vi "PC_Main.vi"() -> ()   [LabVIEW 2020]
doc: "Use this template to build a producer/consumer design pattern with events to produce queue items. Use this design pattern instead of the User Interface Event Handler pattern for user interfaces when you want to execute code asynchronously in response to an event without slowing the user interface responsiveness."
uses:
  <vilib>/userdefined/High Color/nirio_resource_hc.ctl
  Invoked_events.ctl
  <vilib>/FPGAPlugInAG/Dynamic/niLvFpga_Close_Dynamic.vi
  <vilib>/FPGAPlugInAG/cRIO-9040/niLvFpga_Open_cRIO-9040.vi
  <vilib>/rvi/interface/common/dynamic/niFpgaDynamicAddResources.vi
  <vilib>/rvi/interface/nirviCloseFPGA/nirviCloseFPGA.xnode
  <vilib>/rvi/interface/nirviOpenFPGA/nirviOpenFPGA.xnode
  FPGA Bitfiles/depapp_FPGATarget_FPGAmain_WC8wSYHNwdY.lvbitx
  FPGA_main.vi
  <instrlib>/Siglent SDG 1000 5000 800 Series/Siglent SDG 1000 5000 800 Series.lvlib
panel:
  in  "Siglent Channel Control":enum32{"Channel 1", "Channel 2"}(tab)
  in  "Output Channel 1 Button":bool
  in  "Channel 1 Parameters":T1={"Peak-to-Peak Amplitude (V)"=0.1, "Frequency (Hz)"=1000.0, "DC Offset ( V)"=0.0, "Waveform Function (0: Sine)"=enum."Sine"} caption="Cluster"
  in  "Channel 2 Parameters":T1={"Peak-to-Peak Amplitude (V)"=0.1, "Frequency (Hz)"=1000.0, "DC Offset ( V)"=0.0, "Waveform Function (0: Sine)"=enum."Sine"} caption="Cluster"
  in  "Output Channel 2 Button":bool
  in  "resource name":T2
  out "FPGA VI Reference Out":refnum<k20>
  in  "Siglent Resource Name":refnum<visa-resource-name>
  in  "Siglent":bool
  in  "FPGA":bool
  in  "stop":bool
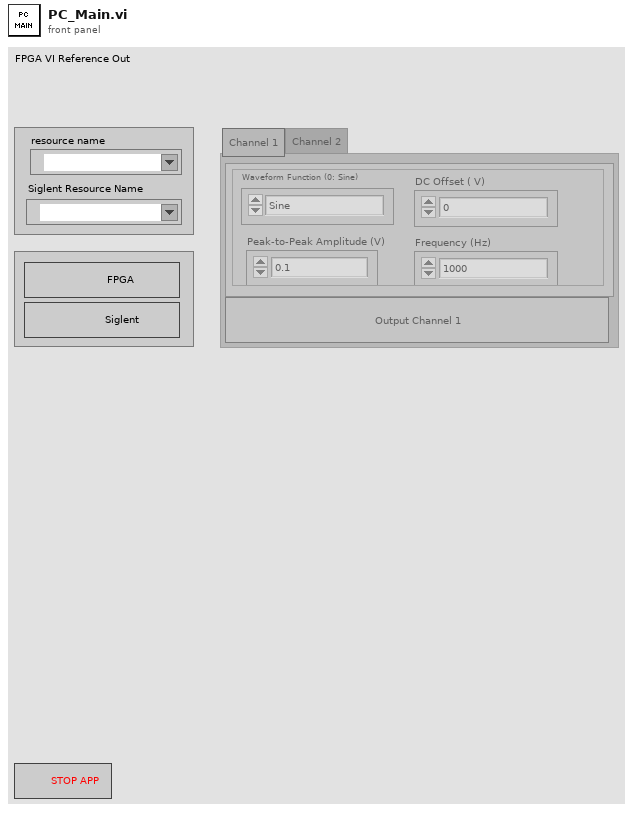
[diagram p1: front panel]
types:
  T1 = cluster{"Peak-to-Peak Amplitude (V)":dbl, "Frequency (Hz)":dbl, "DC Offset ( V)":dbl, "Waveform Function (0: Sine)":enum16{"Sine", "Square", "Triangle", "DC", "Pulse", "Arb"}}
  T2 = typedef "nirio_resource_hc.ctl" = tag
  T3 = typedef "Invoked_events.ctl" = enum16{"Siglent Channel Output Change", "Siglent Channel Parameters Changed", "Stop FPGA", "Initialize FPGA", "Stop Siglent", "Initialize Siglent"}
  T4 = enum8{"Enabled", "Disabled", "Disabled and Grayed Out"}
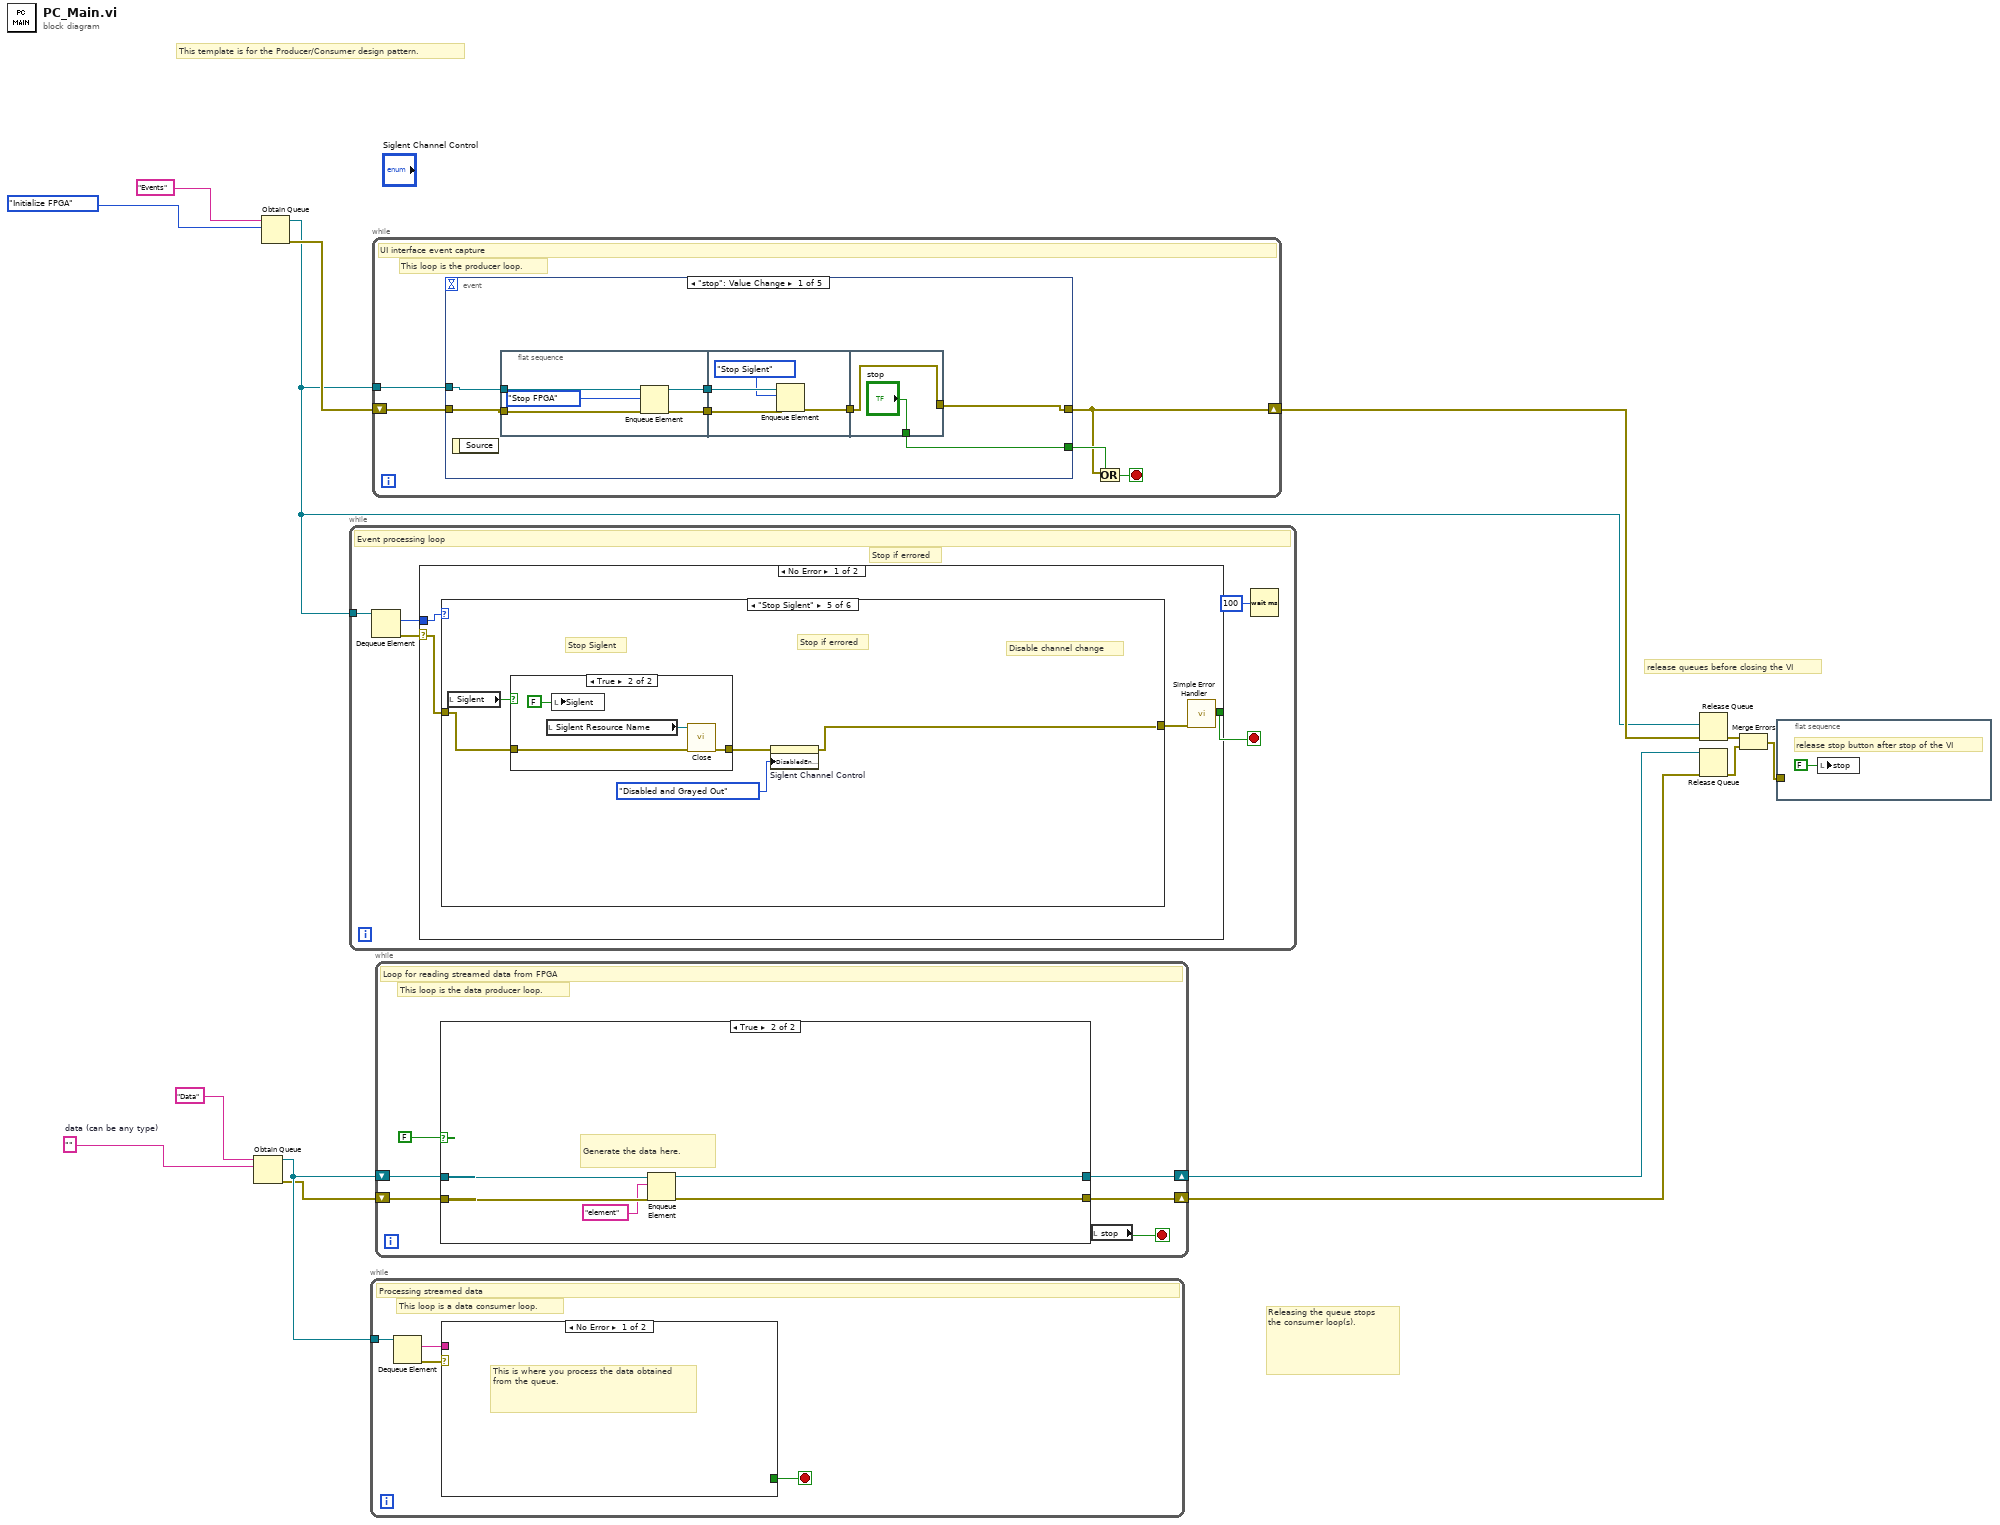
[diagram p0: block diagram]
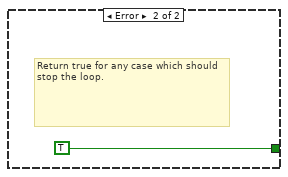
[diagram p2: hidden frame]
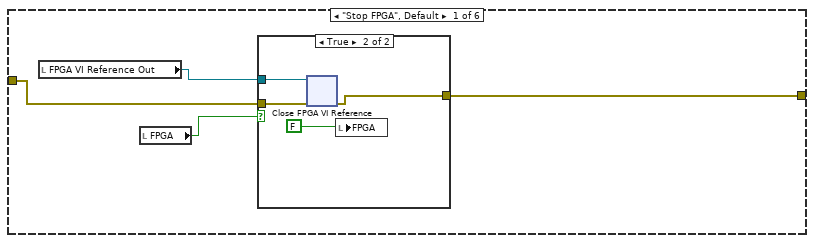
[diagram p4: hidden frame]
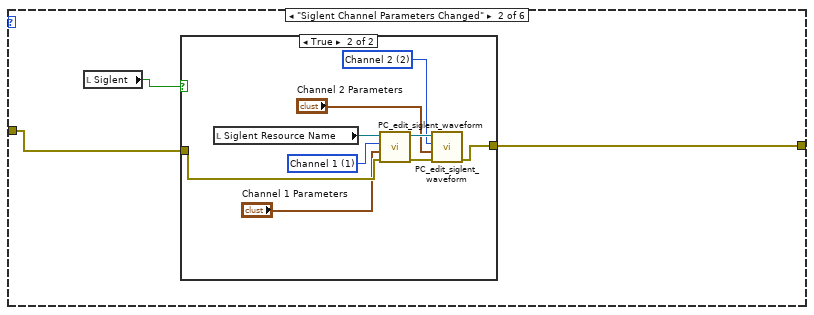
[diagram p6: hidden frame]
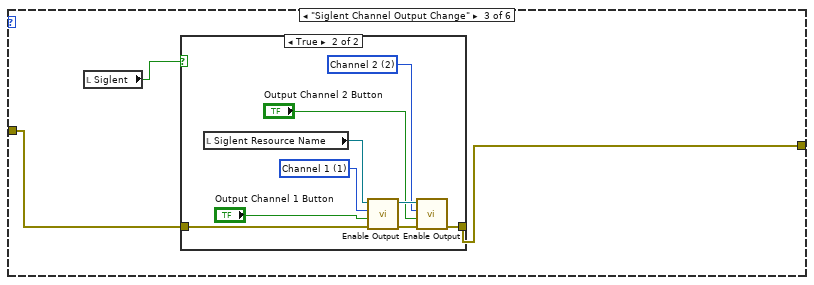
[diagram p8: hidden frame]
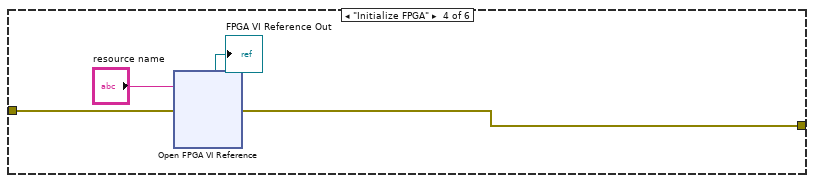
[diagram p10: hidden frame]
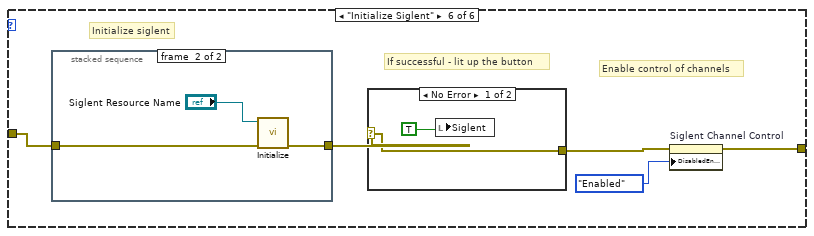
[diagram p12: hidden frame]
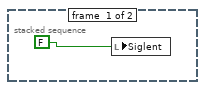
[diagram p13: hidden frame]
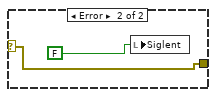
[diagram p14: hidden frame]
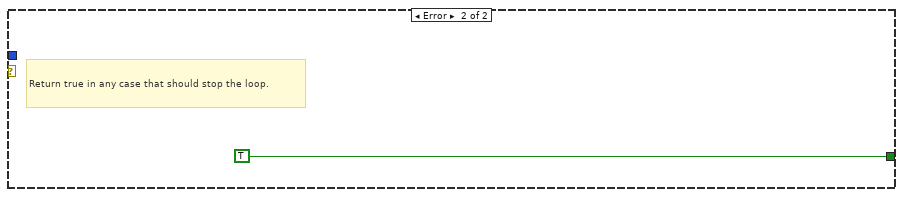
[diagram p15: hidden frame]
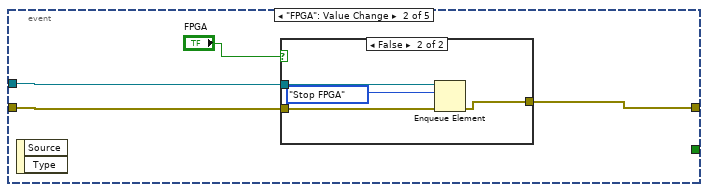
[diagram p16: hidden frame]
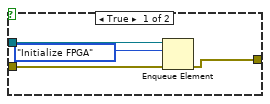
[diagram p17: hidden frame]
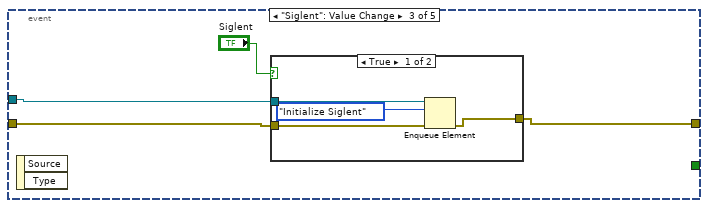
[diagram p18: hidden frame]
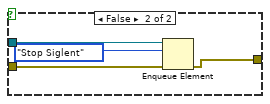
[diagram p19: hidden frame]
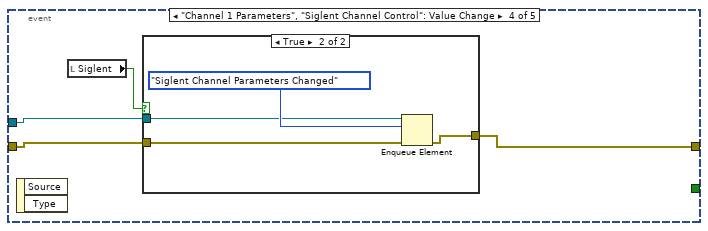
[diagram p20: hidden frame]
diagram:
  w7 = ""  # data (can be any type)
  # "release queues before closing the VI"
  # "Releasing the queue stops the consumer loop(s)."
  # "This template is for the Producer/Consumer design pattern."
  n1 = Obtain Queue(name (unnamed)="Data", element data type=w7) -> (queue out=w11:refnum<queue>, error out=w10:errorcluster)  [unwired: 3 in, 1 out]
  n2 = Obtain Queue(name (unnamed)="Events", element data type=Invoked_events."Initialize FPGA") -> (queue out=w12:refnum<queue>, error out=w14:errorcluster)  [unwired: 3 in, 1 out]
  n3 = while {
    tunnel: w12 -> [w19]
    stop <- w16 stop-if-true
    # "Stop if errored"
    # "Event processing loop"
    n4 = Dequeue Element(queue=w19) -> (element=w17:T3, error out=w18:errorcluster)  [unwired: 2 in, 2 out]
    n5 = case shown="No Error" w18 {
      selector: w18 -> [w21 _]
      tunnel: w17 -> [w22 _]
      tunnel: [_ TRUE] -> w16
      frame No Error {
        n6 = case shown="\"Stop Siglent\"" w22 {
          tunnel: w21 -> [w26 w34 w47 w61 w65 w76]
          tunnel: [w23 w33 w46 w60 w63 w72] -> w20
          frame "Stop FPGA", Default {
            n7 = local read "FPGA VI Reference Out"() -> (w25:refnum<k20>)
            n8 = local read "FPGA"() -> (w24:bool)
            n9 = case shown="True" w24 {
              tunnel: w26 -> [w27 w31]
              tunnel: w25 -> [_ w29]
              tunnel: [w27 w30] -> w23
              frame False {
              }
              frame True {
                n10 = xnode "Close FPGA VI Reference"("FPGA VI Reference In"=w29, "error in"=w31) -> ("error out"=w30:errorcluster)
                n11 = local write "FPGA"(FALSE) -> ()
              }
            }
          }
          frame "Siglent Channel Parameters Changed" {
            n12 = local read "Siglent"() -> (w32:bool)
            n13 = case shown="True" w32 {
              tunnel: w34 -> [w35 w43]
              tunnel: [w35 w36] -> w33
              frame False {
              }
              frame True {
                w37 = 2 items=["Channel 1"=1, "Channel 2"=2] ("Channel (1:Channel 1)")
                w44 = 1 items=["Channel 1"=1, "Channel 2"=2] ("Channel (1:Channel 1)")
                n14 = local read "Siglent Resource Name"() -> (w42:refnum<visa-resource-name>)
                n15 = call "PC_edit_siglent_waveform.vi"("error in (no error)"=w43, "Channel 1 Parameters"="Channel 1 Parameters", "Channel (1:Channel 1)"=w44, "VISA Refnum in"=w42) -> ("error out"=w41:errorcluster, "VISA resource name out"=w40:refnum<visa-resource-name>)  [unwired: 6 in]
                n16 = call "PC_edit_siglent_waveform.vi"("error in (no error)"=w41, "Channel 1 Parameters"="Channel 2 Parameters", "Channel (1:Channel 1)"=w37, "VISA Refnum in"=w40) -> ("error out"=w36:errorcluster)  [unwired: 6 in, 1 out]
              }
            }
          }
          frame "Siglent Channel Output Change" {
            n17 = local read "Siglent"() -> (w45:bool)
            n18 = case shown="True" w45 {
              tunnel: w47 -> [w48 w57]
              tunnel: [w48 w49] -> w46
              frame False {
              }
              frame True {
                w52 = 2 items=["Channel 1"=1, "Channel 2"=2] ("Channel (1:Channel 1)")
                w56 = 1 items=["Channel 1"=1, "Channel 2"=2] ("Channel (1:Channel 1)")
                n19 = local read "Siglent Resource Name"() -> (w55:refnum<visa-resource-name>)
                n20 = call <instrlib>:"Enable Output.vi"("error in (no error)"=w57, "Enable Output (T: Enable)"="Output Channel 1 Button", "Channel (1:Channel 1)"=w56, "VISA resource name"=w55) -> ("error out"=w51:errorcluster, "VISA resource name out"=w54:refnum<visa-resource-name>)  [unwired: 6 in]
                n21 = call <instrlib>:"Enable Output.vi"("error in (no error)"=w51, "Enable Output (T: Enable)"="Output Channel 2 Button", "Channel (1:Channel 1)"=w52, "VISA resource name"=w54) -> ("error out"=w49:errorcluster)  [unwired: 6 in, 1 out]
              }
            }
          }
          frame "Initialize FPGA" {
            n22 = xnode "Open FPGA VI Reference"("error in"=w61, "resource name"="resource name") -> ("FPGA VI Reference Out"=→"FPGA VI Reference Out":refnum<k20>, "error out"=w60:errorcluster)
          }
          frame "Stop Siglent" {
            # "Disable channel change"
            # "Stop if errored"
            # "Stop Siglent"
            n23 = local read "Siglent"() -> (w66:bool)
            n24 = case shown="True" w66 {
              tunnel: w65 -> [w67 w71]
              tunnel: [w67 w69] -> w64
              frame False {
              }
              frame True {
                n25 = local read "Siglent Resource Name"() -> (w70:refnum<visa-resource-name>)
                n26 = local write "Siglent"(FALSE) -> ()
                n27 = call <instrlib>:"Close.vi"("error in (no error)"=w71, "VISA resource name"=w70) -> ("error out"=w69:errorcluster)  [unwired: 9 in]
              }
            }
            n28 = property on="Siglent Channel Control" class="TabCtl (strict)"(error in=w64, "DisabledEnum"=T4."Disabled and Grayed Out" ("Disabled")) -> (error out=w63:errorcluster)  [unwired: 1 in, 1 out]
          }
          frame "Initialize Siglent" {
            # "Enable control of channels"
            # "If successful - lit up the button"
            # "Initialize siglent"
            n29 = stacked-sequence {
              tunnel: w76 -> [_ w79]
              tunnel: [_ w78] -> w75
              frame #0 {
                n30 = local write "Siglent"(FALSE) -> ()
              }
              frame #1 {
                n31 = call <instrlib>:"Initialize.vi"("error in (no error)"=w79, "VISA resource name"="Siglent Resource Name") -> ("error out"=w78:errorcluster)  [unwired: 8 in, 1 out]
              }
            }
            n32 = case shown="No Error" w75 {
              selector: w75 -> [w82 w84]
              tunnel: [w82 w84] -> w73
              frame No Error {
                n33 = local write "Siglent"(TRUE) -> ()
              }
              frame Error {
                n34 = local write "Siglent"(FALSE) -> ()
              }
            }
            n35 = property on="Siglent Channel Control" class="TabCtl (strict)"(error in=w73, "DisabledEnum"=T4."Enabled" ("Disabled")) -> (error out=w72:errorcluster)  [unwired: 1 in, 1 out]
          }
        }
        n36 = call <vilib>:"Simple Error Handler.vi"("error in (no error)"=w20) -> ()  [unwired: 4 in, 5 out]
      }
      frame Error {
        # "Return true in any case that should stop the loop."
      }
    }
    n37 = Wait (ms)(milliseconds to wait=u32 100) -> ()  [unwired: 1 out]
  }
  n38 = while {
    tunnel: w11 -> [w89]
    stop <- w86 stop-if-true
    # "This loop is a data consumer loop."
    # "Processing streamed data"
    n39 = Dequeue Element(queue=w89) -> (element=w87:string, error out=w88:errorcluster)  [unwired: 2 in, 2 out]
    n40 = case shown="No Error" w88 {
      tunnel: w87 -> [_ _]
      tunnel: [_ TRUE] -> w86
      frame No Error {
        # "This is where you process the data obtained from the queue."
      }
      frame Error {
        # "Return true for any case which should stop the loop."
      }
    }
  }
  n41 = while {
    shift-right: [w91] -> w13
    shift-left: w14 -> [w94]
    tunnel: w12 -> [w95]
    stop <- w92 stop-if-true
    # "This loop is the producer loop."
    # "UI interface event capture"
    n42 = event shown="[0] \"stop\": Value Change" {
      selector: _ -> [_ _ _ _ _]
      dyn-events: _ -> [_ _ _ _ _]
      timeout: _ -> [_ _ _ _ _]
      tunnel: w95 -> [w102 w117 w129 w141 w149]
      tunnel: w94 -> [w101 w116 w128 w140 w148]
      tunnel: [w97 w115 w127 w139 w147] -> w91
      tunnel: [w100 _ _ _ _] -> w93
      event "stop": Value Change {
        n43 = event-data() -> ()  [unwired: 1 in, 1 out]
        n44 = flat-sequence {
          tunnel: w102 -> [w107]
          tunnel: w101 -> [w106]
          tunnel: [w104] -> w99
          tunnel: [w103] -> w98
          tunnel: w99 -> [w111]
          tunnel: w98 -> [w110]
          tunnel: [w108] -> w96
          tunnel: ["stop"] -> w100
          tunnel: [w112] -> w97
          tunnel: w96 -> [w112]
          frame #0 {
            n45 = Enqueue Element(queue=w107, element=Invoked_events."Stop FPGA", error in (no error)=w106) -> (queue out=w104:refnum<queue>, error out=w103:errorcluster)  [unwired: 1 in, 1 out]
          }
          frame #1 {
            n46 = Enqueue Element(queue=w111, element=Invoked_events."Stop Siglent", error in (no error)=w110) -> (error out=w108:errorcluster)  [unwired: 1 in, 2 out]
          }
          frame #2 {
          }
        }
      }
      event "FPGA": Value Change {
        n47 = event-data() -> ()  [unwired: 1 in, 2 out]
        n48 = case shown="False" "FPGA" {
          tunnel: w117 -> [w121 w125]
          tunnel: w116 -> [w120 w124]
          tunnel: [w119 w123] -> w115
          frame True {
            n49 = Enqueue Element(queue=w121, element=Invoked_events."Initialize FPGA", error in (no error)=w120) -> (error out=w119:errorcluster)  [unwired: 1 in, 2 out]
          }
          frame False {
            n50 = Enqueue Element(queue=w125, element=Invoked_events."Stop FPGA", error in (no error)=w124) -> (error out=w123:errorcluster)  [unwired: 1 in, 2 out]
          }
        }
      }
      event "Siglent": Value Change {
        n51 = event-data() -> ()  [unwired: 1 in, 2 out]
        n52 = case shown="True" "Siglent" {
          tunnel: w129 -> [w133 w137]
          tunnel: w128 -> [w132 w136]
          tunnel: [w131 w135] -> w127
          frame True {
            n53 = Enqueue Element(queue=w133, element=Invoked_events."Initialize Siglent", error in (no error)=w132) -> (error out=w131:errorcluster)  [unwired: 1 in, 2 out]
          }
          frame False {
            n54 = Enqueue Element(queue=w137, element=Invoked_events."Stop Siglent", error in (no error)=w136) -> (error out=w135:errorcluster)  [unwired: 1 in, 2 out]
          }
        }
      }
      event "Channel 1 Parameters", "Siglent Channel Control": Value Change {
        n55 = event-data() -> ()  [unwired: 1 in, 2 out]
        n56 = local read "Siglent"() -> (w138:bool)
        n57 = case shown="True" w138 {
          tunnel: w141 -> [_ w145]
          tunnel: w140 -> [w142 w144]
          tunnel: [w142 w143] -> w139
          frame False {
          }
          frame True {
            n58 = Enqueue Element(queue=w145, element=Invoked_events."Siglent Channel Parameters Changed", error in (no error)=w144) -> (error out=w143:errorcluster)  [unwired: 1 in, 2 out]
          }
        }
      }
      event "Output Channel 2 Button", "Output Channel 1 Button": Value Change {
        n59 = event-data() -> ()  [unwired: 1 in, 2 out]
        n60 = local read "Siglent"() -> (w150:bool)
        n61 = case shown="True" w150 {
          tunnel: [w151 w154] -> w147
          tunnel: w149 -> [_ w153]
          tunnel: w148 -> [w151 w152]
          frame False {
          }
          frame True {
            n62 = Enqueue Element(queue=w153, element=Invoked_events."Siglent Channel Output Change", error in (no error)=w152) -> (error out=w154:errorcluster)  [unwired: 1 in, 2 out]
          }
        }
      }
    }
    n63 = Or(x=w91, y=w93) -> (x .or. y?=w92:bool)
  }
  n64 = while {
    shift-right: [w158] -> w8
    shift-left: w10 -> [w159]
    shift-right: [w160] -> w9
    shift-left: w11 -> [w161]
    stop <- w156 stop-if-true
    # "This loop is the data producer loop."
    # "Loop for reading streamed data from FPGA"
    n65 = case shown="True" FALSE ("Case Constant\n(See Context Help)") {
      tunnel: w161 -> [w163 w168]
      tunnel: [w163 w167] -> w160
      tunnel: w159 -> [w162 w166]
      tunnel: [w162 w165] -> w158
      frame False {
      }
      frame True {
        # "Generate the data here."
        n66 = Enqueue Element(queue=w168, element="element", error in (no error)=w166) -> (queue out=w167:refnum<queue>, error out=w165:errorcluster)  [unwired: 1 in, 1 out]
      }
    }
    n67 = local read "stop"() -> (w156:bool)
  }
  n68 = Release Queue(queue=w12, error in (no error)=w13) -> (error out=w3:errorcluster)  [unwired: 1 in, 2 out]
  n69 = Release Queue(queue=w9, error in (no error)=w8) -> (error out=w2:errorcluster)  [unwired: 1 in, 2 out]
  n70 = Merge Errors(w3, w2) -> (w1:errorcluster)
  n71 = flat-sequence {
    tunnel: w1 -> [_]
    frame #0 {
      # "release stop button after stop of the VI"
      n72 = local write "stop"(FALSE) -> ()
    }
  }
